vi "correction_move_with_velocity.vi"(0 "Sys_num":i32=1, 1 "Moving Velocity":dbl=1.5, 2 "Final Velocity":dbl=0.1, 3 "No.of digits":i16=4, 4 "step":dbl=0.5, 5 "Conn. Axes":string[](array[string]), 6 "Stop ref":refnum<vi>, 7 "stage_num":i32, 9 "position ref":refnum<vi>, 11 "Stage error in":errorcluster, 12 "Start":dbl=50.0, 13 "Stop":dbl=51.0, 14 "polling time":u32=100) -> (10 "Direction":bool, 15 "Stage error out":errorcluster)   [LabVIEW 2011]
doc: "This vi will move the stage to the desitination, AND the stage approachs the destination from defined direction depending the direction-flag. Step determines the overshoot distance.\nAfter this, the velocity is set to final velocity for further small step measurements."
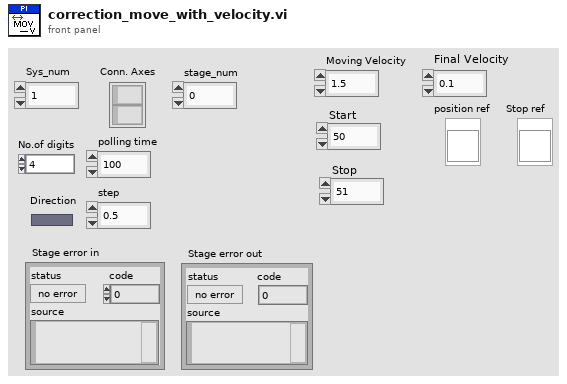
[diagram p1: front panel]
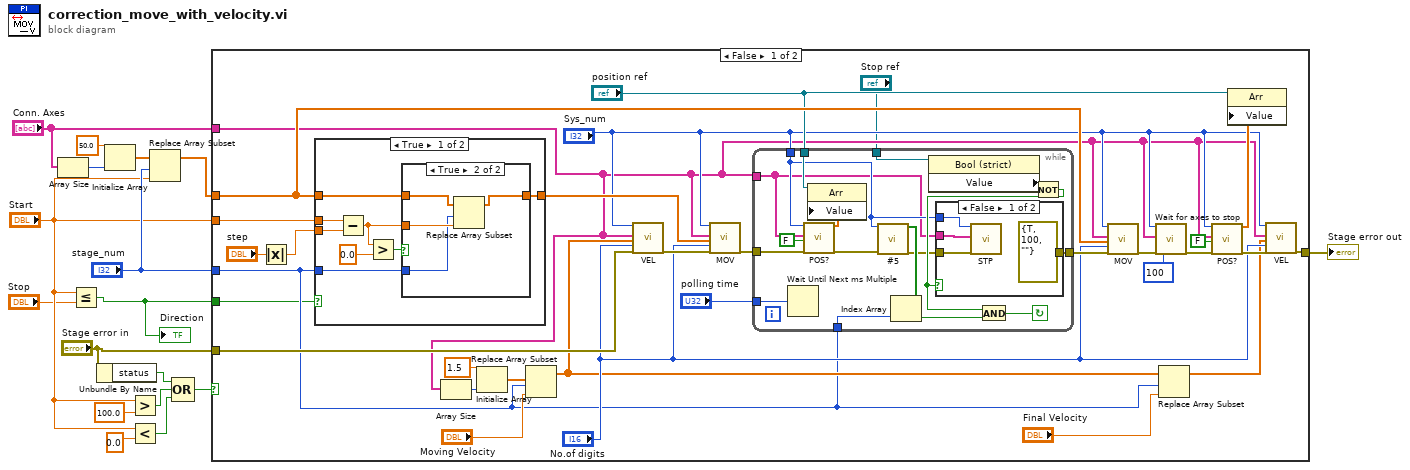
[diagram p0: block diagram]
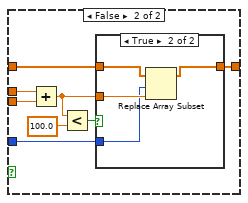
[diagram p4: hidden frame]
diagram:
  n1 = Array Size(array="Conn. Axes") -> (size(s)=w8:i32)
  n2 = Less Or Equal?(x="Start", y="Stop") -> (x <= y?=w1:bool)
  "Direction" <- w1
  n3 = Unbundle By Name("Stage error in") -> ("status"=w14:bool)
  n4 = Initialize Array(50.0 ("element"), w8) -> (w6:dbl[])
  n5 = Greater?(x="Start", y=100.0) -> (0:w12:bool)
  n6 = Less?(x="Start", y=0.0) -> (x < y?=w11:bool)
  n7 = Replace Array Subset(array=w6, new element="Start", index="stage_num") -> (w4:dbl[])
  n8 = Compound Arithmetic op=OR(w14, w12, w11) -> (w13:bool)
  n9 = case shown="False" w13 {
    tunnel: [w30 w97] -> w17
    tunnel: "stage_num" -> [w25 _]
    tunnel: w4 -> [w40 _]
    tunnel: "Start" -> [w46 _]
    tunnel: "Stage error in" -> [w41 w97]
    tunnel: "Conn. Axes" -> [w22 _]
    tunnel: w1 -> [w24 _]
    frame False {
      n10 = Absolute Value(x="step") -> (abs(x)=w47:dbl)
      n11 = case shown="True" w24 {
        tunnel: w46 -> [w78 w91]
        tunnel: w25 -> [w74 w87]
        tunnel: w40 -> [w73 w86]
        tunnel: [w72 w85] -> w36
        tunnel: w47 -> [w71 w84]
        frame True {
          n12 = Subtract(x=w78, y=w71) -> (x-y=w75:dbl)
          n13 = Greater?(x=w75, y=0.0) -> (0:w77:bool)
          n14 = case shown="True" w77 {
            tunnel: w75 -> [_ w83]
            tunnel: w74 -> [_ w82]
            tunnel: w73 -> [w79 w81]
            tunnel: [w79 w80] -> w72
            frame False {
            }
            frame True {
              n15 = Replace Array Subset(array=w81, new element=w83, index=w82) -> (w80:dbl[])
            }
          }
        }
        frame False {
          n16 = Add(x=w91, y=w84) -> (x+y=w88:dbl)
          n17 = Less?(x=w88, y=100.0) -> (x < y?=w90:bool)
          n18 = case shown="True" w90 {
            tunnel: w88 -> [_ w96]
            tunnel: w87 -> [_ w95]
            tunnel: w86 -> [w92 w94]
            tunnel: [w92 w93] -> w85
            frame False {
            }
            frame True {
              n19 = Replace Array Subset(array=w94, new element=w96, index=w95) -> (w93:dbl[])
            }
          }
        }
      }
      n20 = Array Size(array=w22) -> (size(s)=w35:i32)
      n21 = Initialize Array(1.5 ("element"), w35) -> (w33:dbl[])
      n22 = Replace Array Subset(array=w33, new element="Moving Velocity", index=w25) -> (w28:dbl[])
      n23 = call "VEL.vi"("System no."="Sys_num", "Axes to set"=w22, "Velocity values"=w28, "No.of digits"="No.of digits", "error in"=w41) -> ("error out"=w45:errorcluster)  [unwired: 13 in, 1 out]
      n24 = call "MOV.vi"("System no."="Sys_num", "Axes to move"=w22, "Position values"=w36, "No.of digits"="No.of digits", "error in"=w45) -> ("error out"=w44:errorcluster)  [unwired: 14 in]
      n25 = while {
        tunnel: w44 -> [w63]
        tunnel: "polling time" -> [w65]
        tunnel: "Sys_num" -> [w50]
        tunnel: w22 -> [w49]
        tunnel: [w52] -> w42
        tunnel: "position ref" -> [w59]
        tunnel: w25 -> [w58]
        tunnel: "Stop ref" -> [w57]
        stop <- w55 continue-if-true
        n26 = Wait Until Next ms Multiple(millisecond multiple=w65) -> ()  [unwired: 1 out]
        n27 = call "POS?.vi"("System no."=w50, "Axes to query"=w49, "All axes?"=FALSE, "error in"=w63) -> ("Position"=w60:dbl[], "error out"=w62:errorcluster)  [unwired: 14 in]
        n28 = property class="Arr"(reference=w59, "Value"=w60) -> ()  [unwired: 1 in, 2 out]
        n29 = call "#5.vi"("System no."=w50, "error in"=w62) -> ("Axis moving?"=w61:bool[], "error out"=w51:errorcluster)  [unwired: 16 in]
        n30 = Index Array(array=w61, index=w58) -> (element=w56:bool)
        n31 = property class="Bool (strict)"(reference=w57) -> ("Value"=w54:bool)  [unwired: 1 in, 2 out]
        n32 = Not(x=w54) -> (.not. x?=w53:bool)
        n33 = case shown="False" w53 {
          tunnel: [errorcluster {"status"=TRUE, "code"=100, "source"=""} ("error out") w70] -> w52
          tunnel: w51 -> [w68 w70]
          tunnel: w50 -> [w67 _]
          tunnel: w49 -> [w66 _]
          frame False {
            n34 = call "STP.vi"("System no."=w67, "Affected axes?"=w66, "error in"=w68) -> ()  [unwired: 16 in, 1 out]
          }
          frame True {
          }
        }
        n35 = And(x=w53, y=w56) -> (x .and. y?=w55:bool)
      }
      n36 = call "MOV.vi"("System no."="Sys_num", "Axes to move"=w22, "Position values"=w40, "No.of digits"="No.of digits", "error in"=w42) -> ("error out"=w21:errorcluster)  [unwired: 14 in]
      n37 = call "Wait for axes to stop.vi"("System no."="Sys_num", "Axes to wait for"=w22, "error in"=w21, "Polling cycle time, ms"=u32 100) -> ("error out"=w20:errorcluster)  [unwired: 14 in, 1 out]
      n38 = Replace Array Subset(array=w28, new element="Final Velocity", index=w25) -> (w26:dbl[])
      n39 = call "POS?.vi"("System no."="Sys_num", "Axes to query"=w22, "All axes?"=FALSE, "error in"=w20) -> ("Position"=w38:dbl[], "error out"=w31:errorcluster)  [unwired: 14 in]
      n40 = property class="Arr"(reference="position ref", "Value"=w38) -> ()  [unwired: 1 in, 2 out]
      n41 = call "VEL.vi"("System no."="Sys_num", "Axes to set"=w22, "Velocity values"=w26, "No.of digits"="No.of digits", "error in"=w31) -> ("error out"=w30:errorcluster)  [unwired: 13 in, 1 out]
    }
    frame True {
    }
  }
  "Stage error out" <- w17
